vi "Read Status Byte Query.vi"(0 "VISA resource name":refnum<visa-resource-name>, 5 "Timeout (ms)":u32, 11 "error in (no error)":errorcluster) -> (4 "VISA resource name out":refnum<visa-resource-name>, 6 "Status Byte Register":T1, 15 "error out":errorcluster)   [LabVIEW 2020, in "Associated Research 78XX Series.lvlib"]
doc: "Queries the <B>Status Byte</B>. Returns the decimal value of the binary-weighted sum of bits.\n\nEach bit represents a status in the instrument.\n\nEx : When Test passes, BIT 0 is set High giving status \"ALL PASS\"\n\nBIT 0 ,01H,(1) All PASS\nBIT 1 ,02H,(2) FAIL\nBIT 2, 04H,(4) ABORT\nBIT 3, 08H,(8) Process\nBIT 4, 10H,(16) Message Available\nBIT 5, 20H,(32) Standard Event (ESB)\nBIT 6, 40H,(64) Request Service (MSS)\nBIT 7, 80H,(128) Prompt"
uses:
  <instrlib>/Associated Research 78XX Series/Associated Research 78XX Series.lvlib
panel:
  # "BIT 0 ,01H,(1)   All PASS\nBIT 1 ,02H,(2)   FAIL\nBIT 2, 04H,(4)   ABORT\nBIT 3, 08H,(8)   Process\nBIT 4, 10H,(16)  Message Available\nBIT 5, 20H,(32)  Standard Event  (ESB)\nBIT 6, 40H,(64)  Request Service (MSS)\nBIT 7, 80H,(128) Prompt"
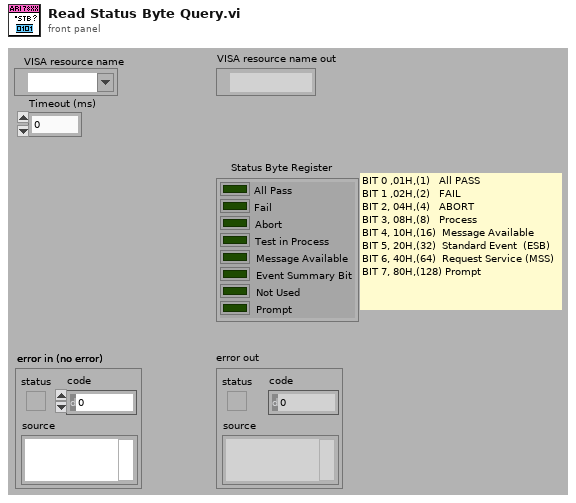
[diagram p1: front panel]
types:
  T1 = cluster{"All Pass":bool, "Fail":bool, "Abort":bool, "Test in Process":bool, "Message Available":bool, "Event Summary Bit":bool, "Not Used":bool, "Prompt":bool}
  T2 = cluster{"Boolean array[0]":bool, "Boolean array[1]":bool, "Boolean array[2]":bool, "Boolean array[3]":bool, "Boolean array[4]":bool, "Boolean array[5]":bool, "Boolean array[6]":bool, "Boolean array[7]":bool}
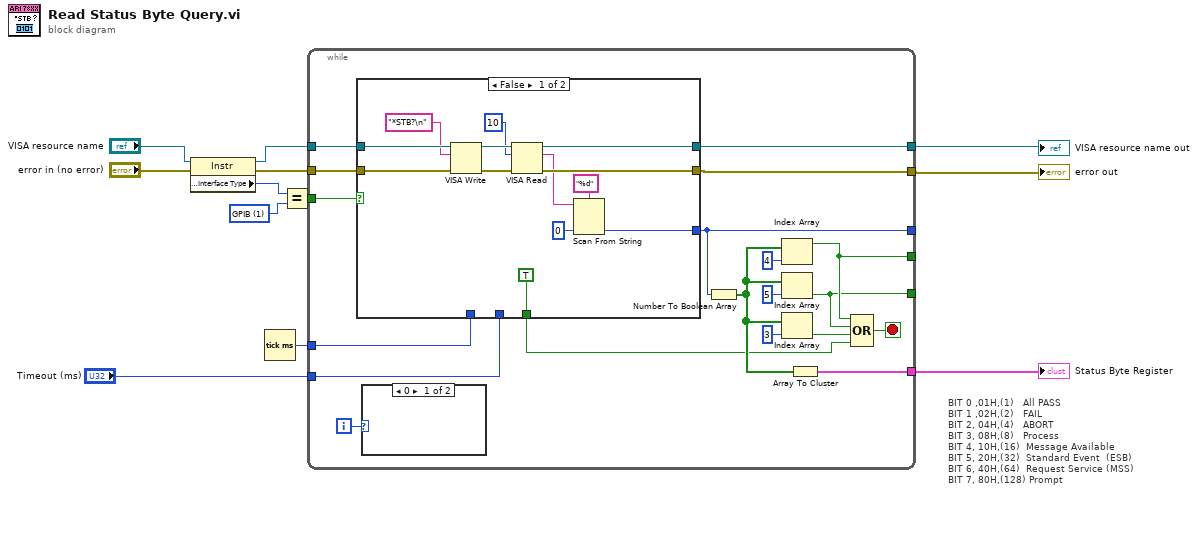
[diagram p0: block diagram]
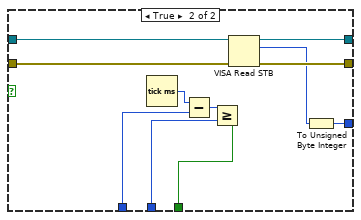
[diagram p2: hidden frame]
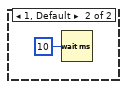
[diagram p3: hidden frame]
diagram:
  w10 = u16 1 items=["GPIB"=1, "VXI"=2, "GPIB-VXI"=3, "Serial"=4, "PXI"=5] ("Interface Information:Interface Type")
  # "BIT 0 ,01H,(1)   All PASS\nBIT 1 ,02H,(2)   FAIL\nBIT 2, 04H,(4)   ABORT\nBIT 3, 08H,(8)   Process\nBIT 4, 10H,(16)  Message Available\nBIT 5, 20H,(32)  Standard Event  (ESB)\nBIT 6, 40H,(64)  Request Service (MSS)\nBIT 7, 80H,(128) Prompt"
  n1 = property class="Instr"(reference="VISA resource name", error in="error in (no error)") -> (reference out=w1:refnum<visa-resource-name>, error out=w2:errorcluster, "Interface Information:Interface Type"=w11:u16)
  n2 = Tick Count (ms)() -> (millisecond timer value=w12:u32)
  n3 = Equal?(x=w11, y=w10) -> (x = y?=w9:bool)
  n4 = while {
    tunnel: w12 -> [w15]
    tunnel: w1 -> [w28]
    tunnel: w2 -> [w27]
    tunnel: w9 -> [w26]
    tunnel: [w24] -> w6
    tunnel: [w23] -> w7
    tunnel: [w22] -> _
    tunnel: [w21] -> _
    tunnel: [w20] -> w5
    tunnel: [w19] -> _
    tunnel: "Timeout (ms)" -> [w14]
    i -> [w25]
    stop <- w29 stop-if-true
    n5 = case shown="False" w26 {
      tunnel: w28 -> [w44 w55]
      tunnel: [w34 w54] -> w23
      tunnel: [w33 w53] -> w24
      tunnel: w27 -> [w43 w52]
      tunnel: [w42 w50] -> w19
      tunnel: w15 -> [_ w47]
      tunnel: w14 -> [_ w46]
      tunnel: [TRUE w45] -> w13
      frame False {
        n6 = VISA Write(VISA resource name=w44, write buffer="*STB?\n" ("Command to Send (empty)"), error in (no error)=w43) -> (VISA resource name out=w36:refnum<visa-resource-name>, error out=w37:errorcluster)  [unwired: 1 out]
        n7 = VISA Read(VISA resource name=w36, byte count=u32 10, error in (no error)=w37) -> (VISA resource name out=w34:refnum<visa-resource-name>, read buffer=w32:string, error out=w33:errorcluster)  [unwired: 1 out]
        n8 = Scan From String(format string="%d" ("Format String"), input string=w32, default 1=u8 0 ("default value 1")) -> (output 1=w42:u8)  [unwired: 2 in, 3 out]
      }
      frame True {
        n9 = Tick Count (ms)() -> (millisecond timer value=w48:u32)
        n10 = Subtract(x=w48, y=w47) -> (x-y=w49:u32)
        n11 = Greater Or Equal?(x=w49, y=w46) -> (x >= y?=w45:bool)
        n12 = VISA Read STB(8:w52, 11:w55) -> (0:w53:errorcluster, 2:w51:u16, 3:w54:refnum<visa-resource-name>)
        n13 = To Unsigned Byte Integer(number=w51) -> (unsigned 8bit integer=w50:u8)
      }
    }
    n14 = case shown="0" w25 {
      frame 0 {
      }
      frame 1, Default {
        n15 = Wait (ms)(milliseconds to wait=u32 10) -> ()  [unwired: 1 out]
      }
    }
    n16 = Number To Boolean Array(number=w19) -> (Boolean array=w17:bool[])
    n17 = Index Array(array=w17, index=4 ("Index")) -> (element=w22:bool)
    n18 = Index Array(array=w17, index=5 ("Index")) -> (element=w21:bool)
    n19 = Index Array(array=w17, index=3 ("Index")) -> (element=w16:bool)
    n20 = Array To Cluster(array=w17) -> (cluster=w20:T2)
    n21 = Compound Arithmetic op=OR(w22, w21, w16, w13) -> (w29:bool)
  }
  "Status Byte Register" <- w5
  "VISA resource name out" <- w7
  "error out" <- w6
